vi "asset.update_set_property.vi"(8 "error in":errorcluster, 11 "AssetUpdateStaging in":refnum<class "AssetUpdateStaging.lvclass">) -> (0 "error out":errorcluster, 3 "AssetUpdateStaging out":refnum<class "AssetUpdateStaging.lvclass">)   [LabVIEW 2020, in "AssetUpdateStaging.lvclass"]
doc: "Sets a property key/value pair that will replace the asset's current properties when the update is applied."
uses:
  AssetUpdateStaging.lvclass
  AssetUpdateStaging.lvclass/AssetUpdateStaging.ctl
  client.lvlib
panel:
  in  "key":string
  in  "value":string
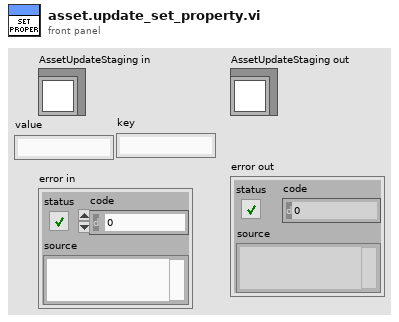
[diagram p1: front panel]
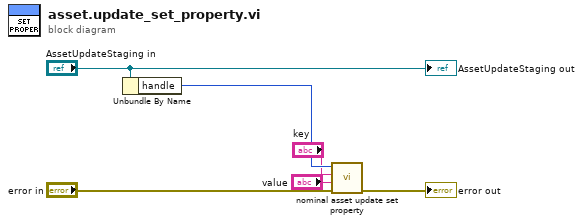
[diagram p0: block diagram]
diagram:
  n1 = Unbundle By Name("AssetUpdateStaging in") -> ("handle"=w4:i32)
  n2 = call "nominal asset update set property.vi"("error in (no error)"="error in", "value"="value", "key"="key", "staging"=w4) -> ("error out"=→"error out":errorcluster)  [unwired: 6 in, 1 out]
  "AssetUpdateStaging out" <- "AssetUpdateStaging in"
